vi "Analysis.Result Summaries, Generate Pareto Per Day.vi"(9 "Type":enum16{"First Pass", "Last Pass", "All"}(ring), 11 "ResultSum":T1[](array[typedef])) -> (3 "FP Pareto":string[][](table))   [LabVIEW 2024]
uses:
  Analysis.Result Summary.ctl
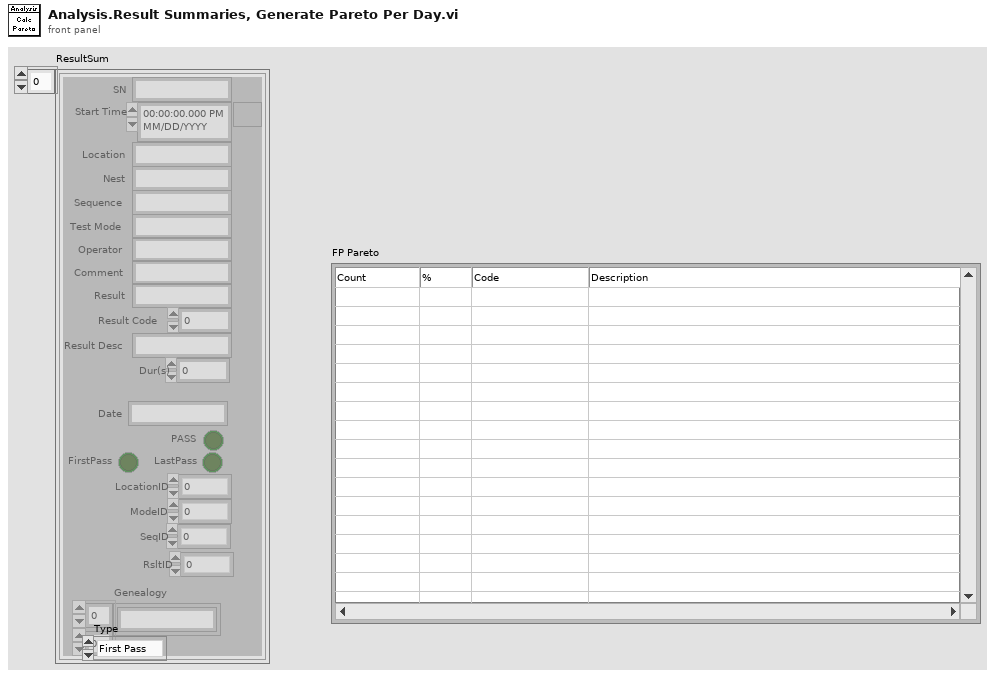
[diagram p1: front panel]
types:
  T1 = typedef "Analysis.Result Summary.ctl" = cluster{"SN":string, "Start Time":timestamp, "Location":string, "Nest":string, "Sequence":string, "Operator":string, "Test Mode":string, "Comment":string, "Result":string, "Result Code":i32, "Result Desc":string, "Date":string, "Dur(s)":dbl, "PASS":bool, "FirstPass":bool, "LastPass":bool, "LocationID":i32, "ModeID":i32, "SeqID":i32, "RsltID":i32, "Genealogy":string[][]}
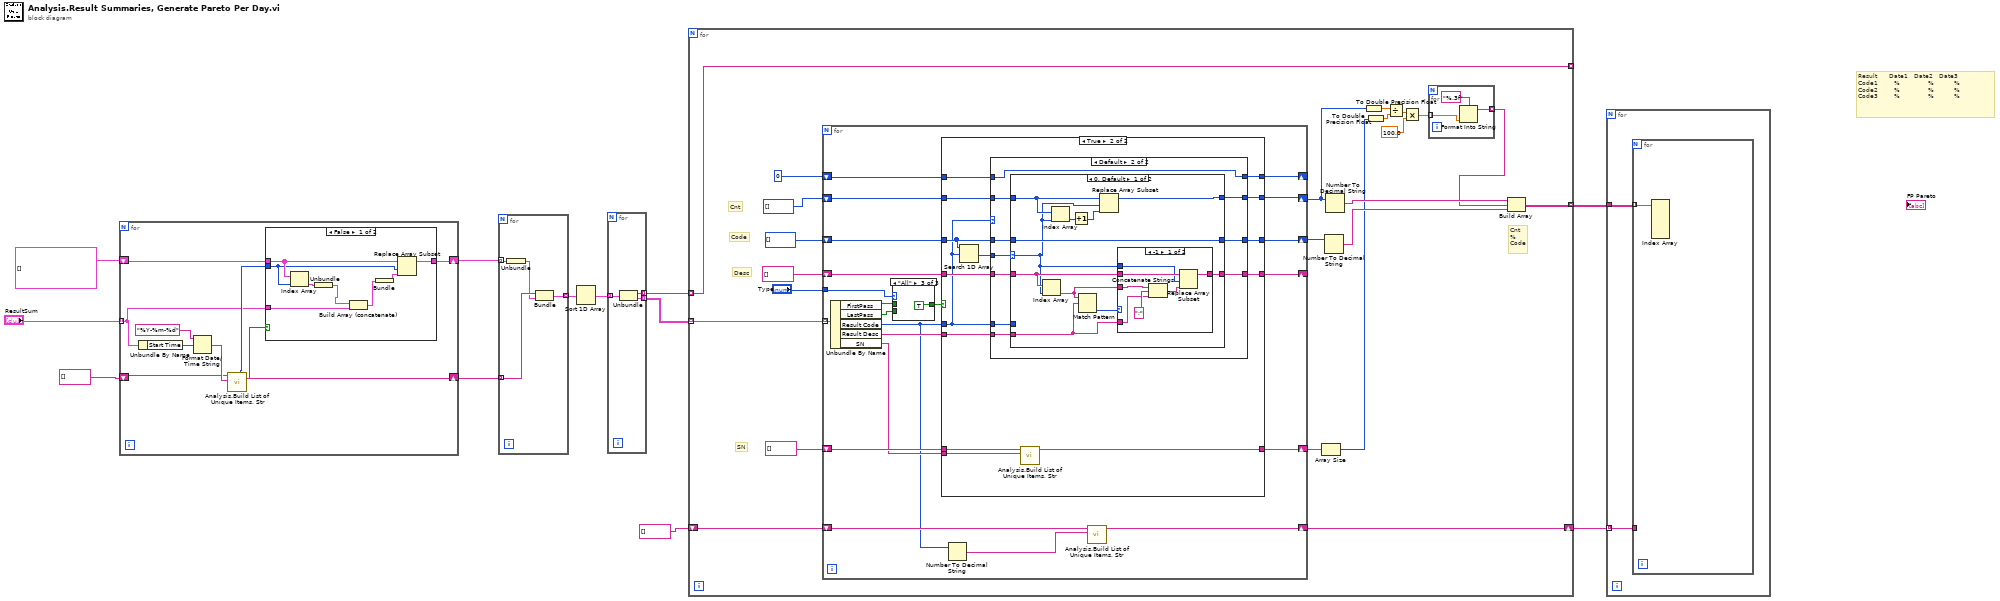
[diagram p0: block diagram]
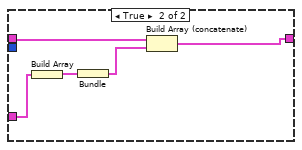
[diagram p2: hidden frame]
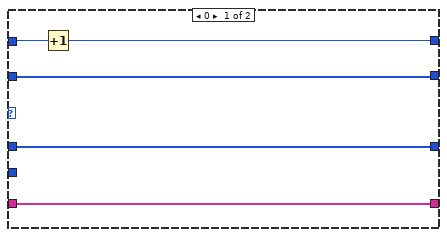
[diagram p6: hidden frame]
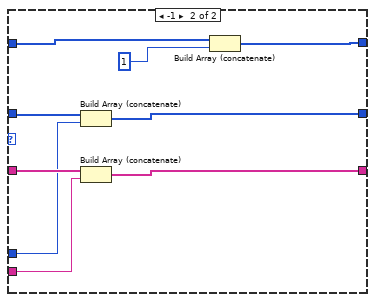
[diagram p8: hidden frame]
diagram:
  # "Result      Date1   Date2   Date3                 \nCode1        %              %          %\nCode2        %              %          %\nCode3        %              %          %"
  n1 = for {
    tunnel: "ResultSum" -> [w16] mode=indexing
    shift-right: [w18] -> w9
    shift-left: string[] [] -> [w19]
    shift-right: [w13] -> w10
    shift-left: cluster{"ResultSum":T1[]}[] [] ("ResultSum") -> [w15]
    n2 = Unbundle By Name(w16) -> ("Start Time"=w22:timestamp)
    n3 = Format Date/Time String(time format string (%c)="%Y-%m-%d", seconds (now)=w22) -> (date/time string=w20:string)  [unwired: 1 in]
    n4 = call "Analysis.Build List of Unique Items, Str.vi"("Item In"=w20, "List In"=w19) -> ("Added"=w14:bool, "List Out"=w18:string[], "Index"=w17:i32)  [unwired: 7 in]
    n5 = case shown="False" w14 {
      tunnel: w17 -> [w29 _]
      tunnel: w16 -> [w28 w33]
      tunnel: w15 -> [w30 w35]
      tunnel: [w23 w34] -> w13
      frame False {
        n6 = Index Array(array=w30, index=w29) -> (element=w27:cluster{"ResultSum":T1[]})
        n7 = Unbundle(w27) -> ("ResultSum"=w26:T1[])
        n8 = Build Array (concatenate)(w26, w28) -> (w25:T1[])
        n9 = Bundle(w25) -> (w24:cluster{T1[]})  [unwired: 1 in]
        n10 = Replace Array Subset(array=w30, new element=w24, index=w29) -> (w23:cluster{"ResultSum":T1[]}[])
      }
      frame True {
        n11 = Build Array(w33) -> (w32:T1[])
        n12 = Bundle(w32) -> (w31:cluster{T1[]})  [unwired: 1 in]
        n13 = Build Array (concatenate)(w35, w31) -> (w34:cluster{"ResultSum":T1[]}[])
      }
    }
  }
  n14 = for {
    tunnel: w10 -> [w37] mode=indexing
    tunnel: w9 -> [w39] mode=indexing
    tunnel: [w38] -> w8 mode=indexing
    n15 = Unbundle(w37) -> ("ResultSum"=w36:T1[])
    n16 = Bundle("String"=w39, "ResultSum"=w36) -> (w38:cluster{"String":string, "ResultSum":T1[]})  [unwired: 1 in]
  }
  n17 = Sort 1D Array(array=w8) -> (sorted array=w7:cluster{"String":string, "ResultSum":T1[]}[])
  n18 = for {
    tunnel: w7 -> [w42] mode=indexing
    tunnel: [w41] -> w6 mode=indexing
    tunnel: [w40] -> w4 mode=indexing
    n19 = Unbundle(w42) -> ("String"=w40:string, "ResultSum"=w41:T1[])
  }
  n20 = for {
    tunnel: w6 -> [w49] mode=indexing
    tunnel: w4 -> [w45] mode=indexing
    tunnel: [w46] -> w2 mode=indexing
    tunnel: [w45] -> _ mode=indexing
    shift-right: [w43] -> w1
    shift-left: string[] [] -> [w44]
    # "Cnt\n%\nCode"
    # "SN"
    # "Desc"
    # "Code"
    # "Cnt"
    n21 = for {
      shift-right: [w86] -> w56
      shift-left: i32[] [] -> [w89]
      shift-right: [w85] -> w53
      shift-left: i32[] [] -> [w88]
      shift-right: [w84] -> _
      shift-left: string[] [] -> [w87]
      tunnel: w49 -> [w81] mode=indexing
      shift-right: [w82] -> _
      shift-left: 0 ("Numeric") -> [w83]
      shift-right: [w77] -> w50
      shift-left: string[] [] -> [w79]
      tunnel: "Type" -> [w76]
      shift-right: [w69] -> w43
      shift-left: w44 -> [w72]
      n22 = Unbundle By Name(w81) -> ("FirstPass"=w75:bool, "LastPass"=w74:bool, "Result Code"=w71:i32, "Result Desc"=w80:string, "SN"=w78:string)
      n23 = case shown="\"All\"" w76 {
        tunnel: w75 -> [w90 _ _]
        tunnel: w74 -> [_ w91 _]
        tunnel: [w90 w91 TRUE] -> w73
        frame "First Pass", Default {
        }
        frame "Last Pass" {
        }
        frame "All" {
        }
      }
      n24 = case shown="True" w73 {
        tunnel: w89 -> [w96 w110]
        tunnel: w88 -> [w95 w109]
        tunnel: w87 -> [w94 w108]
        tunnel: [w96 w107] -> w86
        tunnel: [w95 w106] -> w85
        tunnel: [w94 w105] -> w84
        tunnel: w83 -> [w97 w104]
        tunnel: [w97 w103] -> w82
        tunnel: w71 -> [_ w102]
        tunnel: w80 -> [_ w101]
        tunnel: w79 -> [w93 w100]
        tunnel: w78 -> [_ w99]
        tunnel: [w93 w98] -> w77
        frame False {
        }
        frame True {
          n25 = Search 1D Array(1D array=w109, element=w102) -> (index of element=w111:i32)  [unwired: 1 in]
          n26 = case shown="Default" w102 {
            tunnel: w111 -> [_ w126]
            tunnel: w110 -> [w116 w125]
            tunnel: w109 -> [w115 w124]
            tunnel: w108 -> [w114 w123]
            tunnel: [w116 w122] -> w107
            tunnel: [w115 w121] -> w106
            tunnel: [w114 w120] -> w105
            tunnel: w102 -> [_ w119]
            tunnel: w101 -> [_ w118]
            tunnel: w104 -> [w113 w117]
            tunnel: [w112 w117] -> w103
            frame 0 {
              n27 = Increment(x=w113) -> (x+1=w112:i32)
            }
            frame Default {
              n28 = case shown="0, Default" w126 {
                selector: w126 -> [w127 _]
                tunnel: w125 -> [w136 w151]
                tunnel: w124 -> [w133 w153]
                tunnel: w123 -> [w131 w154]
                tunnel: [w137 w150] -> w122
                tunnel: [w133 w149] -> w121
                tunnel: [w130 w148] -> w120
                tunnel: w119 -> [_ w146]
                tunnel: w118 -> [w128 w147]
                frame 0, Default {
                  n29 = Index Array(array=w131, index=w127) -> (element=w129:string)
                  n30 = Index Array(array=w136, index=w127) -> (element=w135:i32)
                  n31 = Increment(x=w135) -> (x+1=w134:i32)
                  n32 = Match Pattern(string=w129, regular expression=w128) -> (offset past match=w132:i32)  [unwired: 1 in, 3 out]
                  n33 = Replace Array Subset(array=w136, new element=w134, index=w127) -> (w137:i32[])
                  n34 = case shown="-1" w132 {
                    tunnel: w131 -> [w143 w145]
                    tunnel: [w144 w145] -> w130
                    tunnel: w129 -> [w142 _]
                    tunnel: w128 -> [w140 _]
                    tunnel: w127 -> [w138 _]
                    frame -1 {
                      n35 = Concatenate Strings(w142, ";", w140) -> (w139:string)
                      n36 = Replace Array Subset(array=w143, new element=w139, index=w138) -> (w144:string[])
                    }
                    frame Default {
                    }
                  }
                }
                frame -1 {
                  n37 = Build Array (concatenate)(w153, w146) -> (w149:i32[])
                  n38 = Build Array (concatenate)(w154, w147) -> (w148:string[])
                  n39 = Build Array (concatenate)(w151, 1) -> (w150:i32[])
                }
              }
            }
          }
          n40 = call "Analysis.Build List of Unique Items, Str.vi"("Item In"=w99, "List In"=w100) -> ("List Out"=w98:string[])  [unwired: 7 in, 2 out]
        }
      }
      n41 = Number To Decimal String(number=w71) -> (decimal integer string=w70:string)  [unwired: 1 in]
      n42 = call "Analysis.Build List of Unique Items, Str.vi"("Item In"=w70, "List In"=w72) -> ("List Out"=w69:string[])  [unwired: 7 in, 2 out]
    }
    n43 = Array Size(array=w50) -> (size(s)=w48:i32)
    n44 = Number To Decimal String(number=w53) -> (decimal integer string=w52:string[])  [unwired: 1 in]
    n45 = Number To Decimal String(number=w56) -> (decimal integer string=w58:string[])  [unwired: 1 in]
    n46 = To Double Precision Float(number=w56) -> (double precision float=w55:dbl[])
    n47 = To Double Precision Float(number=w48) -> (double precision float=w54:dbl)
    n48 = Divide(x=w55, y=w54) -> (x/y=w59:dbl[])
    n49 = Multiply(x=w59, y=100.0) -> (x*y=w61:dbl[])
    n50 = for {
      tunnel: w61 -> [w67] mode=indexing
      tunnel: [w66] -> w57 mode=indexing
      n51 = Format Into String(format string="%.3f", w67) -> (resulting string=w66:string)  [unwired: 2 in, 1 out]
    }
    n52 = Build Array(w58, w57, w52) -> (w46:string[][])
  }
  n53 = for {
    tunnel: w2 -> [w155]
    tunnel: w1 -> [w156] mode=indexing
    n54 = for {
      tunnel: w156 -> [_]
      tunnel: w155 -> [w157] mode=indexing
      n55 = Index Array(array=w157) -> ()  [unwired: 6 in, 3 out]
    }
  }
